vi "Esercitazione 6 - Media Array.vi"() -> ()   [LabVIEW 2018]
panel:
  out "Media":dbl
  out "Array*Media":dbl[](array[numeric])
  in  "Array":dbl[](array[numeric])
  # "dato un array input di  lunghezza arbitraria, determinare la media aritmetica"
  # "fornire inoltre un array formato dalla media moltiplicata per ciascun elemento\ndell'array iniziale"
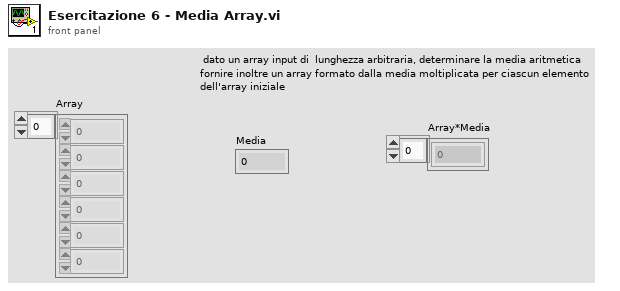
[diagram p1: front panel]
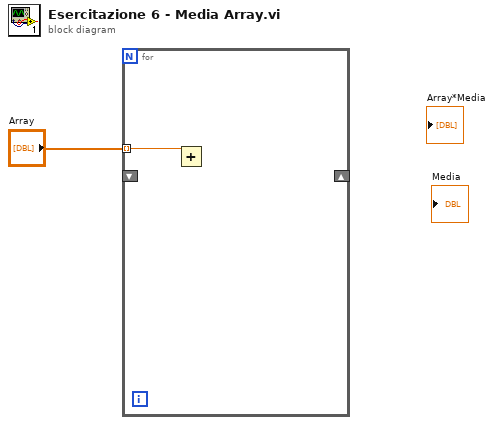
[diagram p0: block diagram]
diagram:
  n1 = for {
    tunnel: "Array" -> [w2] mode=indexing
    shift-right: _ -> [_]
    shift-left: _ -> [_]
    n2 = Add(x=w2) -> ()  [unwired: 1 in, 1 out]
  }
